vi "High G retreival Monitoring GFV..vi"(1 "Action":T1, 5 "Index(0)":i32, 9 "Axis(0 = X , 1 = Y , 2 = Z)":i32, 11 "error in (no error)":errorcluster, 12 "Number items(init. 6000)":i32=6000) -> (3 "fraction complete":dbl, 6 "Index":i32, 10 "Axis":i32, 14 "All retreived":bool, 15 "error out":errorcluster)   [LabVIEW 2010]
uses:
  Gig H retreival monitoror Action.ctl
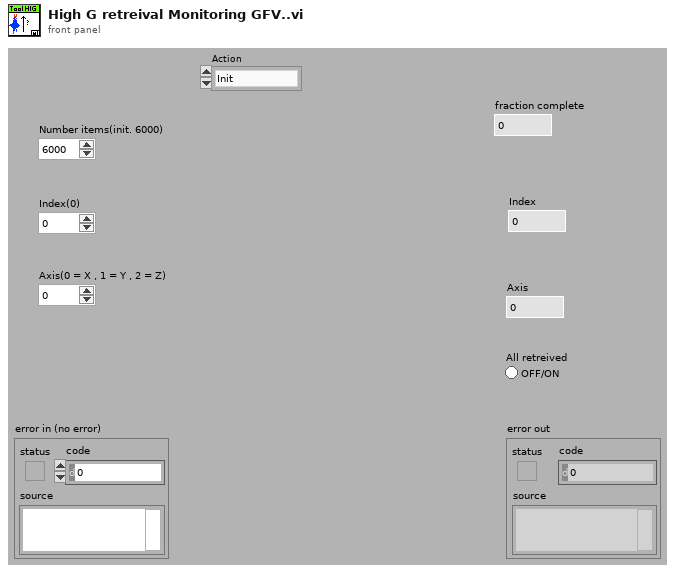
[diagram p1: front panel]
types:
  T1 = typedef "Gig H retreival monitoror Action.ctl" = enum16{"Init", "Get", "Received"}
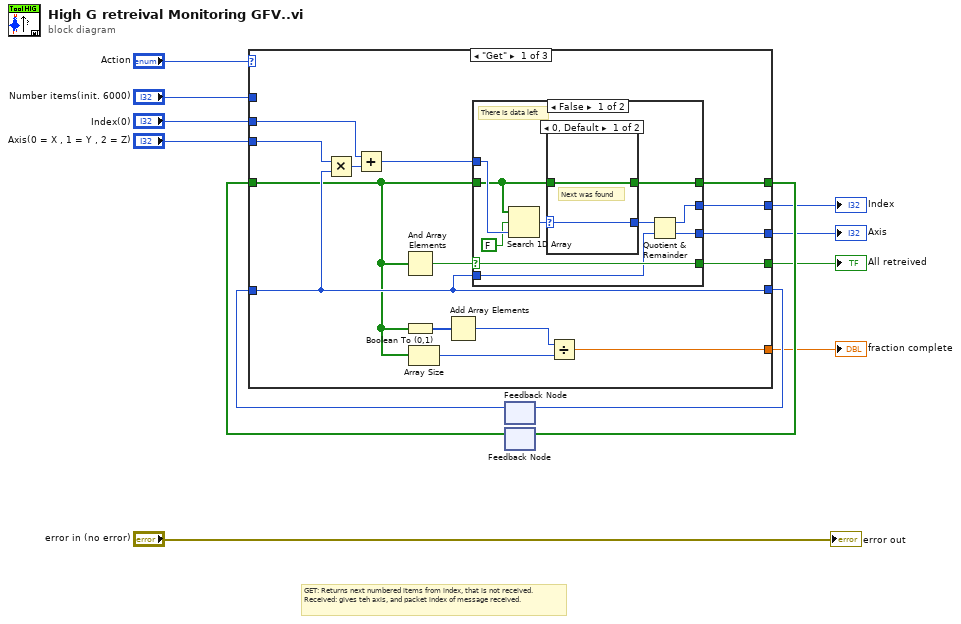
[diagram p0: block diagram]
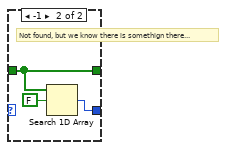
[diagram p2: hidden frame]
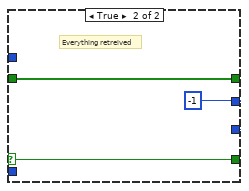
[diagram p3: hidden frame]
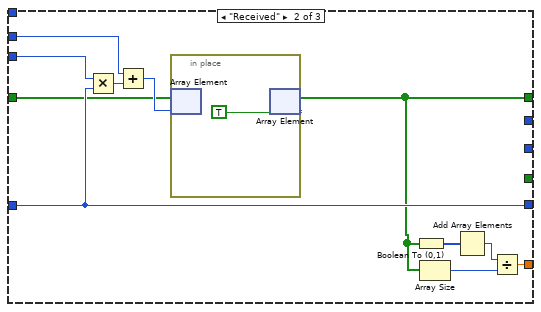
[diagram p4: hidden frame]
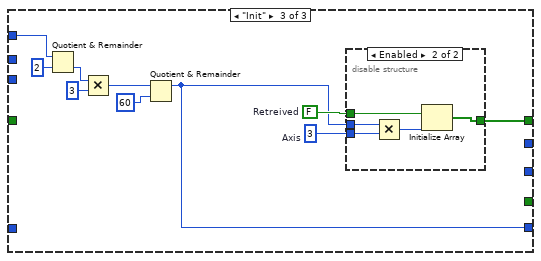
[diagram p5: hidden frame]
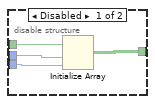
[diagram p6: hidden frame]
diagram:
  # "GET: Returns next numbered items from index, that is not received. \nReceived: gives teh axis, and packet index of message received."
  n1 = feedback #1() -> (w5:i32)  [unwired: 1 in]
  n2 = feedback #2() -> (w10:bool[])  [unwired: 1 in]
  n3 = case shown="\"Get\"" "Action" {
    tunnel: "Number items(init. 6000)" -> [_ _ w63]
    tunnel: [w23 w47 w60] -> w11
    tunnel: w10 -> [w16 w48 _]
    tunnel: "Index(0)" -> [w26 w57 _]
    tunnel: "Axis(0 = X , 1 = Y , 2 = Z)" -> [w27 w54 _]
    tunnel: [w22 _ _] -> w7
    tunnel: [w21 w53 w59] -> w6
    tunnel: w5 -> [w21 w53 _]
    tunnel: [w20 _ _] -> w3
    tunnel: [w19 _ _] -> w4
    tunnel: [w14 w49 _] -> w2
    frame "Get" {
      n4 = Multiply(x=w27, y=w21) -> (x*y=w28:i32)
      n5 = Add(x=w26, y=w28) -> (x+y=w25:i32)
      n6 = And Array Elements(Boolean array=w16) -> (logical AND=w24:bool)
      n7 = Boolean To (0,1)(Boolean=w16) -> (0, 1=w18:i16[])
      n8 = Array Size(array=w16) -> (size(s)=w17:i32)
      n9 = Add Array Elements(numeric array=w18) -> (sum=w15:i16)
      n10 = case shown="False" w24 {
        selector: w24 -> [w37 w45]
        tunnel: w16 -> [w35 w46]
        tunnel: w25 -> [w38 _]
        tunnel: [w36 w46] -> w23
        tunnel: [w37 w45] -> w22
        tunnel: w21 -> [w31 _]
        tunnel: [w30 w44] -> w20
        tunnel: [w29 w44] -> w19
        frame False {
          # "There is data left"
          n11 = Search 1D Array(1D array=w35, element=FALSE, start index (0)=w38) -> (index of element=w33:i32)
          n12 = case shown="0, Default" w33 {
            selector: w33 -> [w39 _]
            tunnel: [w40 w43] -> w36
            tunnel: w35 -> [w40 w43]
            tunnel: [w39 w41] -> w32
            frame 0, Default {
              # "Next was found"
            }
            frame -1 {
              # "Not found, but we know there is somethign there..."
              n13 = Search 1D Array(1D array=w43, element=FALSE) -> (index of element=w41:i32)  [unwired: 1 in]
            }
          }
          n14 = Quotient & Remainder(x=w32, y=w31) -> (x-y*floor(x/y)=w29:i32, floor(x/y)=w30:i32)
        }
        frame True {
          w44 = -1
          # "Everything retreived"
        }
      }
      n15 = Divide(x=w15, y=w17) -> (x/y=w14:dbl)
    }
    frame "Received" {
      n16 = Multiply(x=w54, y=w53) -> (x*y=w55:i32)
      n17 = Add(x=w57, y=w55) -> (x+y=w56:i32)
      n18 = in-place {
        n19 = in-place-array #3(w48, w56) -> ()  [unwired: 1 out]
        n20 = in-place-array #3(TRUE) -> (w47:bool[])  [unwired: 1 out]
      }
      n21 = Boolean To (0,1)(Boolean=w47) -> (0, 1=w52:i16[])
      n22 = Array Size(array=w47) -> (size(s)=w51:i32)
      n23 = Add Array Elements(numeric array=w52) -> (sum=w50:i16)
      n24 = Divide(x=w50, y=w51) -> (x/y=w49:dbl)
    }
    frame "Init" {
      w61 = FALSE  # Retreived
      w62 = 3  # Axis
      n25 = Quotient & Remainder(x=w63, y=2) -> (floor(x/y)=w67:i32)  [unwired: 1 out]
      n26 = Multiply(x=w67, y=3) -> (x*y=w65:i32)
      n27 = Quotient & Remainder(x=w65, y=60) -> (x-y*floor(x/y)=w59:i32)  [unwired: 1 out]
      n28 = disable-structure shown="Enabled" {
        disable-tunnel: w59 -> [w72 w76]
        disable-tunnel: w62 -> [w71 w77]
        disable-tunnel: w61 -> [w70 w75]
        disable-tunnel: [w69 w73] -> w60
        frame Disabled {
          n29 = Initialize Array(w70, w72, w71) -> (w69:bool[][])
        }
        frame Enabled {
          n30 = Multiply(x=w76, y=w77) -> (x*y=w74:i32)
          n31 = Initialize Array(w75, w74) -> (w73:bool[])
        }
      }
    }
  }
  "All retreived" <- w7
  "Index" <- w4
  "Axis" <- w3
  "fraction complete" <- w2
  n32 = feedback-in #1(w6) -> ()
  n33 = feedback-in #2(w11) -> ()
  "error out" <- "error in (no error)"
